vi "Totes to Speed.vi"(11 "Tote#":dbl format="%#_13g") -> (3 "XtraSpeed":dbl)   [LabVIEW 2014]
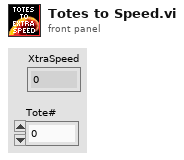
[diagram p1: front panel]
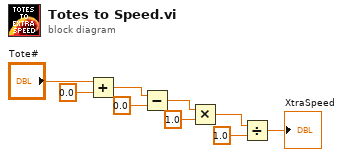
[diagram p0: block diagram]
diagram:
  n1 = Add(x="Tote#", y=0.0) -> (x+y=w4:dbl)
  n2 = Subtract(x=w4, y=0.0) -> (x-y=w3:dbl)
  n3 = Multiply(x=w3, y=1.0) -> (x*y=w2:dbl)
  n4 = Divide(x=w2, y=1.0) -> (x/y=→"XtraSpeed":dbl)
